vi "DSO1K Get Time Automeasure.vi"() -> ()   [LabVIEW 2009]
doc: "<B>This example shows how to get the automeasure parameter as data logger value. </B>"
uses:
  <instrlib>/DSO1K/DSO1K.lvlib
panel:
  in  "Time Measure (0:Frequency)":u16(ring) caption="Time Measurement" items=["Frequency", "Period", "RiseTime", "FallTime", "+Width", "-Width", "Dutycycle", "+Pulses", "-Pulses", "+Edges", "-Edges"]
  in  "Source (1: Channel 1)":u16(ring)=1 items=["Channel 1"=1, "Channel 2"=2, "Channel 3"=3, "Channel 4"=4, "MATH"=5]
  out "Waveform Chart":dbl(graph)
  in  "stop":bool
  in  "Logging Period (500)":u32=500
  in  "VISA resource name":refnum<visa-resource-name>
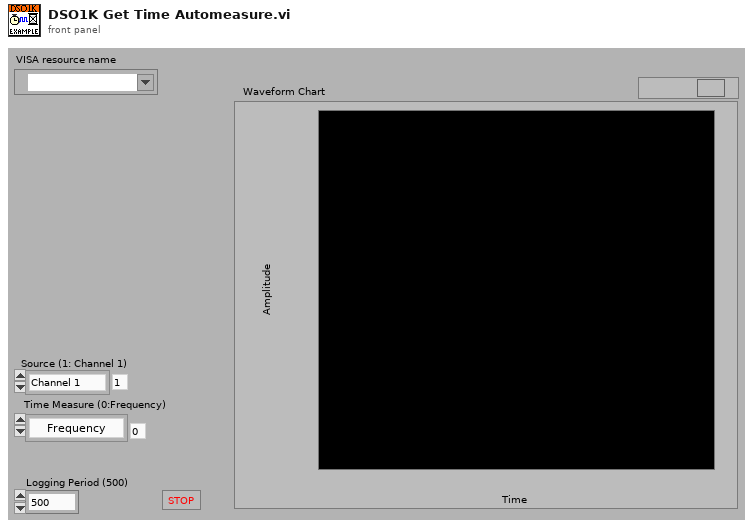
[diagram p1: front panel]
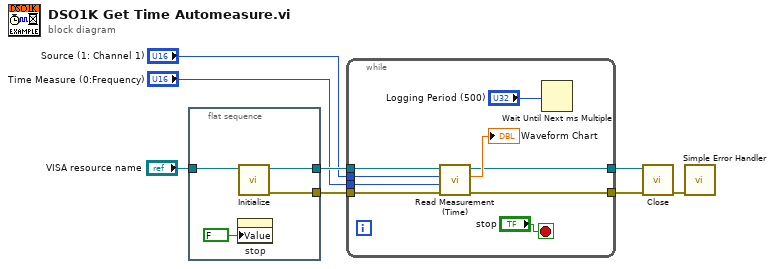
[diagram p0: block diagram]
diagram:
  n1 = flat-sequence {
    tunnel: [w12] -> w7
    tunnel: [w11] -> w6
    tunnel: "VISA resource name" -> [w10]
    frame #0 {
      n2 = property on="stop" class="Bool (strict)"("Value"=FALSE ("stop")) -> ()  [unwired: 2 in, 2 out]
      n3 = call <instrlib>:"Initialize.vi"("VISA resource name"=w10) -> ("error out"=w11:errorcluster, "VISA resource name out"=w12:refnum<visa-resource-name>)  [unwired: 9 in]
    }
  }
  n4 = while {
    tunnel: w7 -> [w15]
    tunnel: w6 -> [w16]
    tunnel: [w18] -> w5
    tunnel: [w17] -> w4
    tunnel: "Time Measure (0:Frequency)" -> [w14]
    tunnel: "Source (1: Channel 1)" -> [w13]
    stop <- "stop" stop-if-true
    n5 = call <instrlib>:"Read Measurement (Time).vi"("error in (no error)"=w16, "Time Measure (0:Frequency)"=w14, "Source (1: Channel 1)"=w13, "VISA resource name"=w15) -> ("error out"=w17:errorcluster, "Time Measurement"=→"Waveform Chart":dbl, "VISA resource name out"=w18:refnum<visa-resource-name>)  [unwired: 5 in]
    n6 = Wait Until Next ms Multiple(millisecond multiple="Logging Period (500)") -> ()  [unwired: 1 out]
  }
  n7 = call <instrlib>:"Close.vi"("error in (no error)"=w4, "VISA resource name"=w5) -> ("error out"=w8:errorcluster)  [unwired: 9 in]
  n8 = call <vilib>:"Simple Error Handler.vi"("error in (no error)"=w8) -> ()  [unwired: 4 in, 5 out]
